vi "Begin.vi"(11 "Image Size":T1=enum."320x240") -> (0 "error out":errorcluster)   [LabVIEW 2012]
doc: "Called before other user functions, this VI is expected to open initial I/O refnums, load in file data, and do all program initialization. Notice that the <B>error out</B> terminal is simply used for data flow. Wiring it to other structures or subVIs ensures that this VI runs first."
uses:
  <vilib>/Rock Robotics/WPI/Camera/WPI_CameraImageSize.ctl
  <vilib>/Rock Robotics/WPI/DriverStation/WPI_DriverStationRobotMode2.ctl
  <vilib>/Rock Robotics/SystemInterfaces/DIO/FPGA_DIOPWMChannel.ctl
  <vilib>/Rock Robotics/WPI/Joystick/WPI_JoystickDeviceEnum.ctl
  <vilib>/Rock Robotics/SystemInterfaces/Typedef/FPGA_TypedefDigitalModule.ctl
  <vilib>/Rock Robotics/WPI/Relay/WPI_RelayDirection.ctl
  <vilib>/Rock Robotics/SystemInterfaces/DIO/FPGA_DIORelayChannel.ctl
  <vilib>/Rock Robotics/SystemInterfaces/AI/FPGA_AIChannel.ctl
  <vilib>/Rock Robotics/SystemInterfaces/AI/FPGA_AIGyroChannel.ctl
  <vilib>/Rock Robotics/SystemInterfaces/DIO/FPGA_DIOChannel.ctl
  <vilib>/Rock Robotics/WPI/Camera/WPI_CameraFrameRate.ctl
  Robot Global Data.vi
  <vilib>/Rock Robotics/WPI/MotorControl/WPI_MotorControlOpen Victor.vi
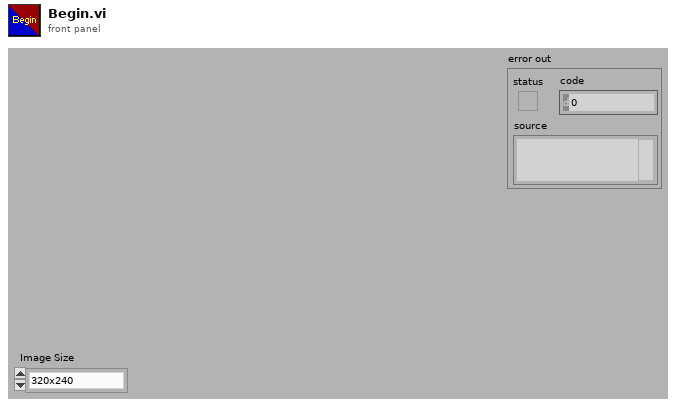
[diagram p1: front panel]
types:
  T1 = typedef "WPI_CameraImageSize.ctl" = enum16{"640x480", "320x240", "160x120"}
  T2 = typedef "FPGA_TypedefDigitalModule.ctl" = enum16{"Digital Module 1", "Digital Module 2"}
  T3 = typedef "FPGA_DIOPWMChannel.ctl" = enum8{"PWM 1", "PWM 2", "PWM 3", "PWM 4", "PWM 5", "PWM 6", "PWM 7", "PWM 8", "PWM 9", "PWM 10", "Invalid"}
  T4 = typedef "FPGA_DIOChannel.ctl" = enum8{"DIO 1", "DIO 2", "DIO 3", "DIO 4", "DIO 5", "DIO 6", "DIO 7", "DIO 8", "DIO 9", "DIO 10", "DIO 11", "DIO 12", "DIO 13", "DIO 14", "Invalid"}
  T5 = typedef "FPGA_DIORelayChannel.ctl" = enum8{"Relay 1", "Relay 2", "Relay 3", "Relay 4", "Relay 5", "Relay 6", "Relay 7", "Relay 8", "Invalid"}
  T6 = typedef "WPI_RelayDirection.ctl" = enum16{"Both directions", "Forward only", "Reverse only"}
  T7 = typedef "WPI_CameraFrameRate.ctl" = u32
  T8 = typedef "FPGA_AIChannel.ctl" = enum8{"AI 1", "AI 2", "AI 3", "AI 4", "AI 5", "AI 6", "AI 7", "AI 8", "Invalid"}
  T9 = typedef "FPGA_AIGyroChannel.ctl" = enum8{"AI 1", "AI 2", "Invalid"}
  T10 = typedef "WPI_JoystickDeviceEnum.ctl" = enum16{"USB 1", "USB 2", "USB 3", "USB 4", "Kinect 1", "Kinect 2"}
  T11 = typedef "WPI_DriverStationRobotMode2.ctl" = enum16{"Autonomous Disabled", "Autonomous Enabled", "Teleop Disabled", "Teleop Enabled", "Timeout", "Finish", "Test Disabled", "Test Enabled"}
  T12 = typedef "WPI_MotorControlDeviceRef.ctl" = cluster{"DeviceStatus":errorcluster, "Type":enum16{"PWM", "CAN"}, "PWM":cluster{"Digital Module":T2, "PWM Channel":T3, "DeadBand":T13}, "CAN":cluster{"Device Number":u8, "Control Mode":T14, "Semaphore":T15, "Max Vout":dbl}, "Invert":bool, "TransformRef":T16, "InvTransformRef":T16}
  T13 = typedef "WPI_PWMDeadband.ctl" = cluster{"Name":string, "maxPositivePwm":i32, "minPositivePwm":i32, "centerPwm":i32, "maxNegativePwm":i32, "minNegativePwm":i32, "angularRange":u16}
  T14 = typedef "WPI_CANJaguar_ControlMode.ctl" = enum8{"Percent VBus", "Current", "Speed", "Position", "Voltage"}
  T15 = typedef "Semaphore RefNum" = refnum<k1>
  T16 = typedef "WPI_PWMTransform_ConPane.ctl" = refnum<vi>
  T17 = typedef "WPI_CameraDevRef.ctl" = cluster{"Camera Address":string, "CameraStatus":errorcluster, "Acquire Image Notifier":refnum<notifier>}
  T18 = typedef "WPI_JoystickDevRef.ctl" = cluster{"Device":T10}
  T19 = typedef "WPI_ServoDeviceRef.ctl" = cluster{"DeviceStatus":errorcluster, "Digital Module":T2, "PWM Channel":T3, "DeadBand":T13}
  T20 = typedef "WPI_RelayDevRef.ctl" = cluster{"DevStatus":errorcluster, "Relay Channel":T5, "Digital Module":T2, "Relay Direction":T6}
  T21 = typedef "WPI_AnalogChannelDevRef.ctl" = cluster{"DevStatus":errorcluster, "Analog Module":T22, "Analog Channel":T8}
  T22 = typedef "FPGA_TypedefAnalogModule.ctl" = enum16{"Analog Module 1", "Analog Module 2"}
  T23 = typedef "WPI_DigitalInputDevRef.ctl" = cluster{"DevStatus":errorcluster, "DIO Channel":T4, "Digital Module":T2}
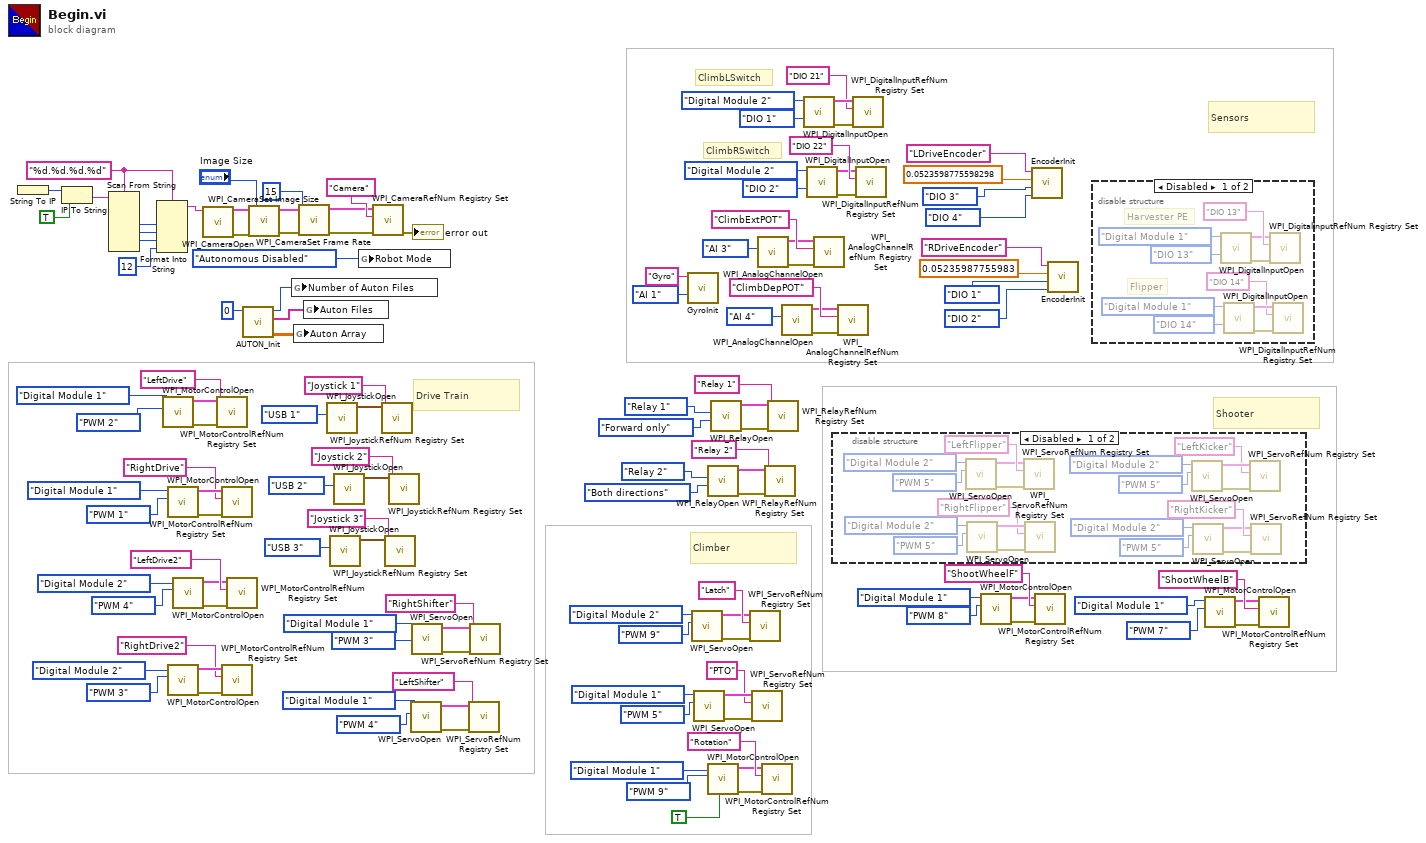
[diagram p0: block diagram]
diagram:
  w40 = "%d.%d.%d.%d" ("format string")
  # "Shooter"
  # "ClimbRSwitch"
  # "ClimbLSwitch"
  # "Drive Train"
  # "Climber"
  # "Sensors"
  n1 = String To IP() -> (0:w47:u32)  [unwired: 1 in]
  n2 = IP To String(1:TRUE ("dot notation? (F)"), 2:w47) -> (0:w45:string)
  n3 = Scan From String(format string=w40, input string=w45) -> (output 1=w44:i32, output 2=w43:i32, output 3=w42:i32)  [unwired: 7 in, 3 out]
  n4 = Format Into String(format string=w40, w44, w43, w42, 12 ("Compression")) -> (resulting string=w39:string)  [unwired: 2 in, 1 out]
  n5 = call-poly <vilib>:"WPI_MotorControlOpen.vi"("PWM Channel"=FPGA_DIOPWMChannel."PWM 2", "Digital Module (Module 1)"=FPGA_TypedefDigitalModule."Digital Module 1") -> ("error out"=w115:errorcluster, "MotorControlDeviceRef"=w116:T12)  [unwired: 8 in]
  n6 = call-poly <vilib>:"WPI_MotorControlOpen.vi"("PWM Channel"=FPGA_DIOPWMChannel."PWM 1", "Digital Module (Module 1)"=FPGA_TypedefDigitalModule."Digital Module 1") -> ("error out"=w122:errorcluster, "MotorControlDeviceRef"=w121:T12)  [unwired: 8 in]
  n7 = call-poly <vilib>:"WPI_MotorControlOpen.vi"("PWM Channel"=FPGA_DIOPWMChannel."PWM 3", "Digital Module (Module 1)"=FPGA_TypedefDigitalModule."Digital Module 2") -> ("error out"=w104:errorcluster, "MotorControlDeviceRef"=w103:T12)  [unwired: 8 in]
  n8 = call-poly <vilib>:"WPI_MotorControlOpen.vi"("PWM Channel"=FPGA_DIOPWMChannel."PWM 4", "Digital Module (Module 1)"=FPGA_TypedefDigitalModule."Digital Module 2") -> ("error out"=w95:errorcluster, "MotorControlDeviceRef"=w96:T12)  [unwired: 8 in]
  n9 = call <vilib>:"WPI_CameraOpen.vi"("Camera Address"=w39) -> ("error out"=w38:errorcluster, "CameraDevRef"=w37:T17)  [unwired: 1 in, 8 out]
  n10 = call <vilib>:"WPI_MotorControlRefNum Registry Set.vi"("error in (no error)"=w115, "refnum name"="LeftDrive", "MotorControlDevRef"=w116) -> ()  [unwired: 7 in, 2 out]
  n11 = call <vilib>:"WPI_MotorControlRefNum Registry Set.vi"("error in (no error)"=w122, "refnum name"="RightDrive", "MotorControlDevRef"=w121) -> ()  [unwired: 7 in, 2 out]
  n12 = call <vilib>:"WPI_MotorControlRefNum Registry Set.vi"("error in (no error)"=w104, "refnum name"="RightDrive2", "MotorControlDevRef"=w103) -> ()  [unwired: 7 in, 2 out]
  n13 = call <vilib>:"WPI_MotorControlRefNum Registry Set.vi"("error in (no error)"=w95, "refnum name"="LeftDrive2", "MotorControlDevRef"=w96) -> ()  [unwired: 7 in, 2 out]
  n14 = call "AUTON_Init.vi"("Default File"=0) -> ("Auton Array"=w123:dbl[][], "Auton Files"=w124:string[], "Number of Auton Files"=w125:i64)  [unwired: 8 in]
  n15 = call <vilib>:"WPI_CameraSet Image Size.vi"("error in (no error)"=w38, "Image Size"="Image Size", "CameraDevRef"=w37) -> ("error out"=w35:errorcluster, "CameraDevRef Out"=w36:T17)  [unwired: 7 out]
  n16 = global write "Robot Global Data.vi" "Number of Auton Files"(w125) -> ()
  n17 = global write "Robot Global Data.vi" "Auton Array"(w123) -> ()
  n18 = call <vilib>:"WPI_CameraSet Frame Rate.vi"("error in (no error)"=w35, "Frame Rate (fps)"=T7 15, "CameraDevRef"=w36) -> ("error out"=w34:errorcluster, "CameraDevRef Out"=w33:T17)  [unwired: 7 out]
  n19 = global write "Robot Global Data.vi" "Auton Files"(w124) -> ()
  n20 = call <vilib>:"WPI_JoystickOpen.vi"("JoystickDevice"=WPI_JoystickDeviceEnum."USB 1") -> ("JoystickDevRef"=w106:T18)  [unwired: 10 in]
  n21 = call <vilib>:"WPI_JoystickOpen.vi"("JoystickDevice"=WPI_JoystickDeviceEnum."USB 3") -> ("JoystickDevRef"=w112:T18)  [unwired: 10 in]
  n22 = call <vilib>:"WPI_JoystickOpen.vi"("JoystickDevice"=WPI_JoystickDeviceEnum."USB 2") -> ("JoystickDevRef"=w111:T18)  [unwired: 10 in]
  n23 = global write "Robot Global Data.vi" "Robot Mode"(WPI_DriverStationRobotMode2."Autonomous Disabled" ("Robot Mode")) -> ()
  n24 = call <vilib>:"WPI_CameraRefNum Registry Set.vi"("error in (no error)"=w34, "refnum name"="Camera", "CameraDevRef"=w33) -> ("error out"=→"error out":errorcluster)  [unwired: 8 out]
  n25 = call <vilib>:"WPI_JoystickRefNum Registry Set.vi"("refnum name"="Joystick 1", "JoystickDevRef"=w106) -> ()  [unwired: 8 in, 2 out]
  n26 = call <vilib>:"WPI_JoystickRefNum Registry Set.vi"("refnum name"="Joystick 3", "JoystickDevRef"=w112) -> ()  [unwired: 8 in, 2 out]
  n27 = call <vilib>:"WPI_JoystickRefNum Registry Set.vi"("refnum name"="Joystick 2", "JoystickDevRef"=w111) -> ()  [unwired: 8 in, 2 out]
  n28 = call <vilib>:"WPI_ServoOpen.vi"("PWM Channel"=FPGA_DIOPWMChannel."PWM 4", "Digital Module (Module 1)"=FPGA_TypedefDigitalModule."Digital Module 1") -> ("error out"=w88:errorcluster, "ServoDeviceRef"=w81:T19)  [unwired: 8 in]
  n29 = call <vilib>:"WPI_ServoOpen.vi"("PWM Channel"=FPGA_DIOPWMChannel."PWM 3", "Digital Module (Module 1)"=FPGA_TypedefDigitalModule."Digital Module 1") -> ("error out"=w87:errorcluster, "ServoDeviceRef"=w86:T19)  [unwired: 8 in]
  n30 = call <vilib>:"WPI_ServoRefNum Registry Set.vi"("error in (no error)"=w88, "refnum name"="LeftShifter", "ServoDeviceRef"=w81) -> ()  [unwired: 7 in, 2 out]
  n31 = call <vilib>:"WPI_ServoRefNum Registry Set.vi"("error in (no error)"=w87, "refnum name"="RightShifter", "ServoDeviceRef"=w86) -> ()  [unwired: 7 in, 2 out]
  n32 = call "GyroInit.vi"("refnum name"="Gyro", "Analog Channel"=FPGA_AIGyroChannel."AI 1") -> ()  [unwired: 8 in]
  n33 = call <vilib>:"WPI_ServoOpen.vi"("PWM Channel"=FPGA_DIOPWMChannel."PWM 9", "Digital Module (Module 1)"=FPGA_TypedefDigitalModule."Digital Module 2") -> ("error out"=w12:errorcluster, "ServoDeviceRef"=w13:T19)  [unwired: 8 in]
  n34 = call <vilib>:"WPI_ServoOpen.vi"("PWM Channel"=FPGA_DIOPWMChannel."PWM 5", "Digital Module (Module 1)"=FPGA_TypedefDigitalModule."Digital Module 1") -> ("error out"=w66:errorcluster, "ServoDeviceRef"=w65:T19)  [unwired: 8 in]
  n35 = call <vilib>:"WPI_RelayOpen.vi"("Relay Direction"=WPI_RelayDirection."Both directions", "Relay Channel"=FPGA_DIORelayChannel."Relay 2") -> ("error out"=w89:errorcluster, "RelayDevRef"=w90:T20)  [unwired: 8 in]
  n36 = call-poly <vilib>:"WPI_MotorControlOpen.vi"("Invert"=TRUE, "PWM Channel"=FPGA_DIOPWMChannel."PWM 9", "Digital Module (Module 1)"=FPGA_TypedefDigitalModule."Digital Module 1") -> ("error out"=w71:errorcluster, "MotorControlDeviceRef"=w70:T12)  [unwired: 7 in]
  n37 = call <vilib>:"WPI_RelayOpen.vi"("Relay Direction"=WPI_RelayDirection."Forward only", "Relay Channel"=FPGA_DIORelayChannel."Relay 1") -> ("error out"=w30:errorcluster, "RelayDevRef"=w29:T20)  [unwired: 8 in]
  n38 = call <vilib>:"WPI_ServoRefNum Registry Set.vi"("error in (no error)"=w12, "refnum name"="Latch", "ServoDeviceRef"=w13) -> ()  [unwired: 7 in, 2 out]
  n39 = call <vilib>:"WPI_ServoRefNum Registry Set.vi"("error in (no error)"=w66, "refnum name"="PTO", "ServoDeviceRef"=w65) -> ()  [unwired: 7 in, 2 out]
  n40 = call <vilib>:"WPI_AnalogChannelOpen.vi"("Analog Channel"=FPGA_AIChannel."AI 3") -> ("error out"=w50:errorcluster, "AIDeviceRef"=w51:T21)  [unwired: 9 in]
  n41 = call <vilib>:"WPI_MotorControlRefNum Registry Set.vi"("error in (no error)"=w71, "refnum name"="Rotation", "MotorControlDevRef"=w70) -> ()  [unwired: 7 in, 2 out]
  n42 = call <vilib>:"WPI_RelayRefNum Registry Set.vi"("error in (no error)"=w89, "refnum name"="Relay 2", "RelayDevRef"=w90) -> ()  [unwired: 7 in, 2 out]
  n43 = call <vilib>:"WPI_RelayRefNum Registry Set.vi"("error in (no error)"=w30, "refnum name"="Relay 1", "RelayDevRef"=w29) -> ()  [unwired: 7 in, 2 out]
  n44 = call <vilib>:"WPI_AnalogChannelOpen.vi"("Analog Channel"=FPGA_AIChannel."AI 4") -> ("error out"=w75:errorcluster, "AIDeviceRef"=w76:T21)  [unwired: 9 in]
  n45 = call <vilib>:"WPI_DigitalInputOpen.vi"("DIO Channel"=FPGA_DIOChannel."DIO 1", "Digital Module (Module 1)"=FPGA_TypedefDigitalModule."Digital Module 2") -> ("error out"=w17:errorcluster, "DigitalInputDevRef"=w18:T23)  [unwired: 8 in]
  n46 = call <vilib>:"WPI_DigitalInputOpen.vi"("DIO Channel"=FPGA_DIOChannel."DIO 2", "Digital Module (Module 1)"=FPGA_TypedefDigitalModule."Digital Module 2") -> ("error out"=w24:errorcluster, "DigitalInputDevRef"=w23:T23)  [unwired: 8 in]
  n47 = call <vilib>:"WPI_AnalogChannelRefNum Registry Set.vi"("error in (no error)"=w50, "refnum name"="ClimbExtPOT", "AIDeviceRef"=w51) -> ()  [unwired: 7 in, 2 out]
  n48 = disable-structure shown="Disabled" {
    frame Disabled {
      n49 = call <vilib>:"WPI_ServoOpen.vi"("PWM Channel"=FPGA_DIOPWMChannel."PWM 5", "Digital Module (Module 1)"=FPGA_TypedefDigitalModule."Digital Module 2") -> ("error out"=w143:errorcluster, "ServoDeviceRef"=w144:T19)  [unwired: 8 in]
      n50 = call <vilib>:"WPI_ServoOpen.vi"("PWM Channel"=FPGA_DIOPWMChannel."PWM 5", "Digital Module (Module 1)"=FPGA_TypedefDigitalModule."Digital Module 2") -> ("error out"=w142:errorcluster, "ServoDeviceRef"=w141:T19)  [unwired: 8 in]
      n51 = call <vilib>:"WPI_ServoRefNum Registry Set.vi"("error in (no error)"=w143, "refnum name"="LeftFlipper", "ServoDeviceRef"=w144) -> ()  [unwired: 7 in, 2 out]
      n52 = call <vilib>:"WPI_ServoRefNum Registry Set.vi"("error in (no error)"=w142, "refnum name"="RightFlipper", "ServoDeviceRef"=w141) -> ()  [unwired: 7 in, 2 out]
      n53 = call <vilib>:"WPI_ServoOpen.vi"("PWM Channel"=FPGA_DIOPWMChannel."PWM 5", "Digital Module (Module 1)"=FPGA_TypedefDigitalModule."Digital Module 2") -> ("error out"=w133:errorcluster, "ServoDeviceRef"=w132:T19)  [unwired: 8 in]
      n54 = call <vilib>:"WPI_ServoOpen.vi"("PWM Channel"=FPGA_DIOPWMChannel."PWM 5", "Digital Module (Module 1)"=FPGA_TypedefDigitalModule."Digital Module 2") -> ("error out"=w128:errorcluster, "ServoDeviceRef"=w134:T19)  [unwired: 8 in]
      n55 = call <vilib>:"WPI_ServoRefNum Registry Set.vi"("error in (no error)"=w133, "refnum name"="LeftKicker", "ServoDeviceRef"=w132) -> ()  [unwired: 7 in, 2 out]
      n56 = call <vilib>:"WPI_ServoRefNum Registry Set.vi"("error in (no error)"=w128, "refnum name"="RightKicker", "ServoDeviceRef"=w134) -> ()  [unwired: 7 in, 2 out]
    }
    frame Enabled {
    }
  }
  n57 = call <vilib>:"WPI_AnalogChannelRefNum Registry Set.vi"("error in (no error)"=w75, "refnum name"="ClimbDepPOT", "AIDeviceRef"=w76) -> ()  [unwired: 7 in, 2 out]
  n58 = call <vilib>:"WPI_DigitalInputRefNum Registry Set.vi"("error in (no error)"=w17, "refnum name"="DIO 21", "DigitalInputDevRef"=w18) -> ()  [unwired: 7 in, 2 out]
  n59 = call <vilib>:"WPI_DigitalInputRefNum Registry Set.vi"("error in (no error)"=w24, "refnum name"="DIO 22", "DigitalInputDevRef"=w23) -> ()  [unwired: 7 in, 2 out]
  n60 = call-poly <vilib>:"WPI_MotorControlOpen.vi"("PWM Channel"=FPGA_DIOPWMChannel."PWM 8", "Digital Module (Module 1)"=FPGA_TypedefDigitalModule."Digital Module 1") -> ("error out"=w7:errorcluster, "MotorControlDeviceRef"=w8:T12)  [unwired: 8 in]
  n61 = call "EncoderInit.vi"("refnum name"="LDriveEncoder", "DistancePerCount"=0.0523598775598298, "DIO Channel"=FPGA_DIOChannel."DIO 3", "DIO Channel 2"=FPGA_DIOChannel."DIO 4") -> ()  [unwired: 7 in]
  n62 = call <vilib>:"WPI_MotorControlRefNum Registry Set.vi"("error in (no error)"=w7, "refnum name"="ShootWheelF", "MotorControlDevRef"=w8) -> ()  [unwired: 7 in, 2 out]
  n63 = call "EncoderInit.vi"("refnum name"="RDriveEncoder", "DistancePerCount"=0.05235987755983, "DIO Channel"=FPGA_DIOChannel."DIO 1", "DIO Channel 2"=FPGA_DIOChannel."DIO 2") -> ()  [unwired: 7 in]
  n64 = disable-structure shown="Disabled" {
    frame Disabled {
      # "Flipper"
      # "Harvester PE"
      n65 = call <vilib>:"WPI_DigitalInputOpen.vi"("DIO Channel"=FPGA_DIOChannel."DIO 13", "Digital Module (Module 1)"=FPGA_TypedefDigitalModule."Digital Module 1") -> ("error out"=w156:errorcluster, "DigitalInputDevRef"=w155:T23)  [unwired: 8 in]
      n66 = call <vilib>:"WPI_DigitalInputOpen.vi"("DIO Channel"=FPGA_DIOChannel."DIO 14", "Digital Module (Module 1)"=FPGA_TypedefDigitalModule."Digital Module 1") -> ("error out"=w149:errorcluster, "DigitalInputDevRef"=w150:T23)  [unwired: 8 in]
      n67 = call <vilib>:"WPI_DigitalInputRefNum Registry Set.vi"("error in (no error)"=w156, "refnum name"="DIO 13", "DigitalInputDevRef"=w155) -> ()  [unwired: 7 in, 2 out]
      n68 = call <vilib>:"WPI_DigitalInputRefNum Registry Set.vi"("error in (no error)"=w149, "refnum name"="DIO 14", "DigitalInputDevRef"=w150) -> ()  [unwired: 7 in, 2 out]
    }
    frame Enabled {
    }
  }
  n69 = call-poly <vilib>:"WPI_MotorControlOpen.vi"("PWM Channel"=FPGA_DIOPWMChannel."PWM 7", "Digital Module (Module 1)"=FPGA_TypedefDigitalModule."Digital Module 1") -> ("error out"=w3:errorcluster, "MotorControlDeviceRef"=w2:T12)  [unwired: 8 in]
  n70 = call <vilib>:"WPI_MotorControlRefNum Registry Set.vi"("error in (no error)"=w3, "refnum name"="ShootWheelB", "MotorControlDevRef"=w2) -> ()  [unwired: 7 in, 2 out]
